vi "Relative Pose.vi"(10 "Final":T1, 11 "Initial":T1) -> (3 "Relative Pose":T1)   [LabVIEW 2019]
uses:
  Typedef/Pose2d.ctl
  Typedef/Translation2d.ctl
  Typedef/Rotation2d.ctl
  <vilib>/Analysis/NI_AALBase.lvlib
  <vilib>/Analysis/baseanly.llb/Real Inverse Matrix.vi
  <vilib>/Analysis/baseanly.llb/Real A x B.vi
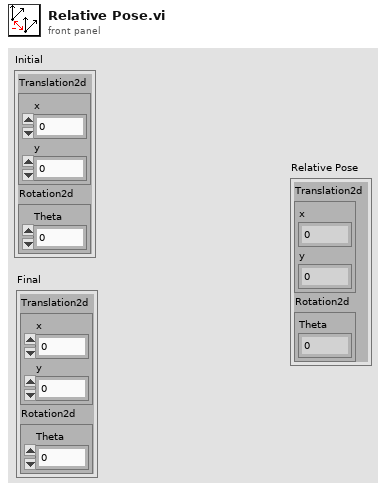
[diagram p1: front panel]
types:
  T1 = typedef "Pose2d.ctl" = cluster{"Translation2d":T2, "Rotation2d":T3}
  T2 = typedef "Translation2d.ctl" = cluster{"x":dbl, "y":dbl}
  T3 = typedef "Rotation2d.ctl" = cluster{"Theta":dbl}
  T4 = typedef "NI_Matrix.lvlib/RealMatrix.ctl" = dbl[][]
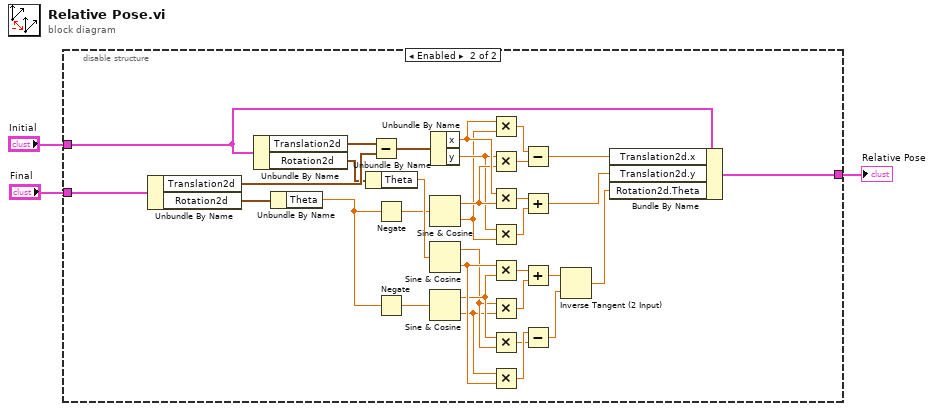
[diagram p0: block diagram]
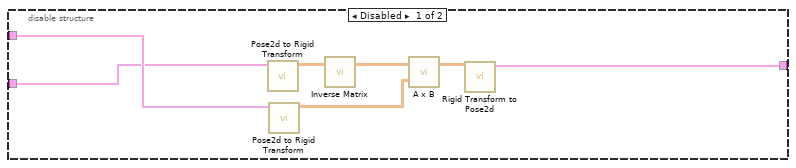
[diagram p2: hidden frame]
diagram:
  n1 = disable-structure shown="Enabled" {
    disable-tunnel: "Initial" -> [w10 w11]
    disable-tunnel: "Final" -> [w9 w12]
    disable-tunnel: [w7 w13] -> w1
    frame Disabled {
      n2 = call "Pose2d to Rigid Transform.vi"("Pose2d"=w9) -> ("Rigid Transform"=w6:T4)  [unwired: 10 in]
      n3 = call "Pose2d to Rigid Transform.vi"("Pose2d"=w10) -> ("Rigid Transform"=w4:T4)  [unwired: 10 in]
      n4 = call-poly <vilib>:"Inverse Matrix.vi"("Input Matrix"=w6) -> ("Inverse Matrix"=w5:T4)  [unwired: 1 in, 1 out]
      n5 = call-poly <vilib>:"A x B.vi"("B"=w4, "A"=w5) -> ("A x B"=w8:T4)  [unwired: 1 out]
      n6 = call "Rigid Transform to Pose2d.vi"("A x B"=w8) -> ("Relative Pose"=w7:T1)  [unwired: 10 in]
    }
    frame Enabled {
      n7 = Unbundle By Name(w12) -> ("Translation2d"=w42:T2, "Rotation2d"=w16:T3)
      n8 = Unbundle By Name(w11) -> ("Translation2d"=w43:T2, "Rotation2d"=w28:T3)
      n9 = Unbundle By Name(w16) -> ("Theta"=w40:dbl)
      n10 = Unbundle By Name(w28) -> ("Theta"=w39:dbl)
      n11 = Subtract(x=w43, y=w42) -> (x-y=w41:T2)
      n12 = Negate(x=w40) -> (-x=w27:dbl)
      n13 = Negate(x=w40) -> (-x=w14:dbl)
      n14 = Sine & Cosine(0:w27) -> (1:w22:dbl, 2:w17:dbl)
      n15 = Sine & Cosine(0:w39) -> (1:w34:dbl, 2:w36:dbl)
      n16 = Sine & Cosine(0:w14) -> (1:w35:dbl, 2:w33:dbl)
      n17 = Unbundle By Name(w41) -> ("x"=w23:dbl, "y"=w18:dbl)
      n18 = Multiply(x=w23, y=w17) -> (x*y=w26:dbl)
      n19 = Multiply(x=w18, y=w22) -> (x*y=w25:dbl)
      n20 = Multiply(x=w23, y=w22) -> (x*y=w21:dbl)
      n21 = Multiply(x=w18, y=w17) -> (x*y=w20:dbl)
      n22 = Multiply(x=w36, y=w35) -> (x*y=w32:dbl)
      n23 = Multiply(x=w34, y=w33) -> (x*y=w31:dbl)
      n24 = Multiply(x=w35, y=w34) -> (x*y=w37:dbl)
      n25 = Multiply(x=w33, y=w36) -> (x*y=w38:dbl)
      n26 = Subtract(x=w26, y=w25) -> (x-y=w24:dbl)
      n27 = Add(x=w21, y=w20) -> (x+y=w19:dbl)
      n28 = Add(x=w32, y=w31) -> (x+y=w29:dbl)
      n29 = Subtract(x=w38, y=w37) -> (x-y=w30:dbl)
      n30 = Inverse Tangent (2 Input)(1:w30, 2:w29) -> (0:w15:dbl)
      n31 = Bundle By Name(cluster=w11, "Translation2d.x"=w24, "Translation2d.y"=w19, "Rotation2d.Theta"=w15) -> (w13:T1)
    }
  }
  "Relative Pose" <- w1
